vi "bh3_ECG_waveform_format.vi"(11 "ECG Waveform Packet":u8[](array[numeric]) format="%02x") -> (2 "ECG data":u32[](array[numeric]), 3 "counter":u8, 4 "milliseconds":u32, 5 "month":u8, 6 "day":u8, 7 "year":u16)   [LabVIEW 2013]
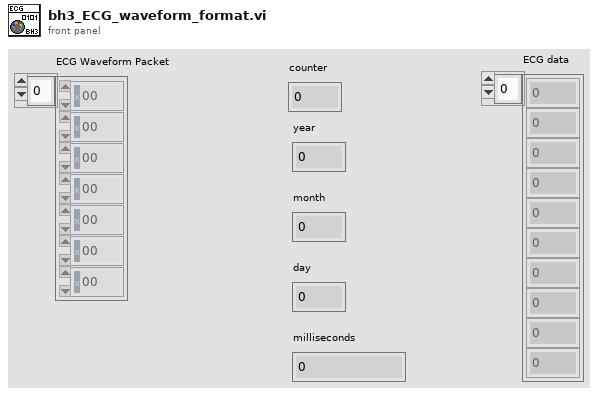
[diagram p1: front panel]
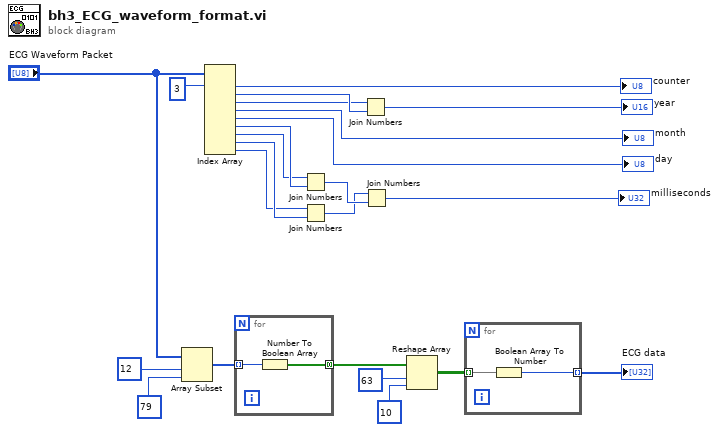
[diagram p0: block diagram]
diagram:
  n1 = Array Subset(array="ECG Waveform Packet", index=12, length=79 ("index")) -> (w1:u8[])
  n2 = Index Array(array="ECG Waveform Packet", index #1=3 ("index")) -> (element #1=→"counter":u8, element #2=w23:u8, element #3=w22:u8, element #4=→"month":u8, element #5=→"day":u8, element #6=w16:u8, element #7=w15:u8, element #8=w12:u8, element #9=w11:u8)  [unwired: 8 in]
  n3 = for {
    tunnel: w1 -> [w25] mode=indexing
    tunnel: [w24] -> w5 mode=concatenating
    n4 = Number To Boolean Array(number=w25) -> (Boolean array=w24:bool[])
  }
  n5 = Join Numbers(hi=w15, lo=w16) -> ((hi.lo)=w14:u16)
  n6 = Join Numbers(hi=w11, lo=w12) -> ((hi.lo)=w13:u16)
  n7 = Join Numbers(hi=w22, lo=w23) -> ((hi.lo)=→"year":u16)
  n8 = Join Numbers(hi=w13, lo=w14) -> ((hi.lo)=→"milliseconds":u32)
  n9 = Reshape Array(w5, 63 ("dimension size"), 10 ("dimension size")) -> (w2:bool[][])
  n10 = for {
    tunnel: w2 -> [w27] mode=indexing
    tunnel: [w26] -> w6 mode=indexing
    n11 = Boolean Array To Number(Boolean array=w27) -> (number=w26:u32)
  }
  "ECG data" <- w6
